vi "Set CurrSensor Record.vi"(8 "error in (no error)":errorcluster, 10 "CurrSensor":T1 {"last updated" format="%<%H:%M\n%d/%m/%Y>T"}, 11 "Main in":refnum<class "Main.lvclass">) -> (0 "error out":errorcluster, 3 "Main out":refnum<class "Main.lvclass">)   [LabVIEW 2019, in "Main.lvclass"]
uses:
  Main.lvclass
  Common/DataTypes/Sensor ranges--cluster.ctl
  Common/DataTypes/Sensor LUT--cluster.ctl
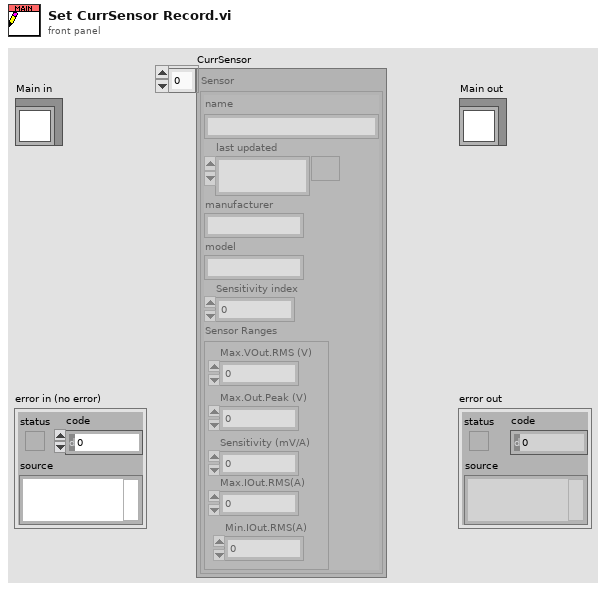
[diagram p1: front panel]
types:
  T1 = typedef "Sensor LUT--cluster.ctl" = cluster{"name":string, "last updated":timestamp, "manufacturer":string, "model":string, "Sensitivity index":dbl, "Sensor Ranges":T2}[]
  T2 = typedef "Sensor ranges--cluster.ctl" = cluster{"Max.VOut.RMS (V)":dbl, "Max.Out.Peak (V)":dbl, "Sensitivity (mV/A)":dbl, "Max.IOut.RMS(A)":dbl, "Min.IOut.RMS(A)":dbl}
  T3 = typedef "Main.lvclass/ObjData--cluster.ctl" = cluster{"Settings":T4, "Public Events":T7, "Dependency":T8, "ReadData-placeholder":T9, "VISA-placeholder":refnum<visa-resource-name>, "InverterWaveformsQ":T10, "Application.TerminateProcess Event":refnum<user-event>, "RawDaqDataQ":T11, "MeasSettings":T12, "InverterDataAcqMode":T13, "DAQState Data":T14, "Private Events":T16, "InvWfmsQ-DT":T10, "DPAuxDataQ":T17, "ProcessingState":T18, "InverterInfo":T19, "CurrInverters":T20[], "InverterLUT Dict":T24, "ESR Chart Ref":refnum<vi>[], "StoreESR BLine Ref":refnum<vi>, "UseSavedESR BLine Ref":refnum<vi>, "CurrSensor":T1}
  T4 = typedef "Main.lvclass/Settings--cluster.ctl" = cluster{"Simulation":bool, "Signal scaling":T5[], "ESR scaling":T6[], "num readings to average":i32[], "ESR alarm threshhold (%)":i32[], "UseDummyVrms":bool, "Dummy Vrms":dbl, "Inverter Database File":path, "default Inverter (name)":string[], "Minimum Current Threshold ":dbl[], "Sensors Database File":path, "default Sensors (name)":string[]}
  T5 = typedef "Main.lvclass/Gain control.ctl" = cluster{"Iin ripple gain":dbl, "Iout ripple gain":dbl, "Iout 60Hz gain ":dbl, "Vout 60Hz gain ":dbl, "Iin ripple offest":dbl, "Iout ripple offset":dbl, "Iout 60Hz offset":dbl, "Vout 60Hz offset":dbl}
  T6 = typedef "Main.lvclass/ESR scaling--cluster.ctl" = cluster{"Gain":dbl, "Offset":dbl}
  T7 = typedef "Main.lvclass/Public Events--cluster.ctl" = cluster{"Main.AsyncCmd Event":refnum<user-event>, "Main.AsyncMsg Event":refnum<user-event>, "stop process":refnum<user-event>, "UpdateControlValue Ev":refnum<user-event>, "ProcessingStateChg Ev":refnum<user-event>}
  T8 = typedef "Main.lvclass/Dependency--cluster.ctl" = cluster{"Config":refnum<class "Config.lvclass">, "DAQ":refnum<class "DAQ_Engine.lvclass">, "Log_Engine":refnum<class "Log_Engine.lvclass">}
  T9 = typedef "Main.lvclass/Read Data--cluster.ctl" = cluster{"Data":dbl}
  T10 = typedef "InverterWaveforms--QRef.ctl" = refnum<queue>
  T11 = typedef "RawDAQDataQRef--cluster.ctl" = refnum<queue>
  T12 = typedef "Measurement Config--cluster.ctl" = cluster{"Data Rate 9775":dbl, "Data Rate 9215":dbl, "Samples RMS 9215":u32, "Samples RMS 9775":u32}
  T13 = typedef "Acquisition Mode--cluster.ctl" = enum16{"3phase", "Single"}
  T14 = typedef "DAQ_Engine.lvclass/DAQStateEvData--cluster.ctl" = cluster{"DAQState":T15, "vData":variant}
  T15 = typedef "DAQState--enum.ctl" = enum16{"Unknown", "Stopped", "Running", "Error"}
  T16 = typedef "Main.lvclass/Private Events--cluster.ctl" = cluster{"PrivateAsync Ev":refnum<user-event>}
  T17 = typedef "DataProcAuxDat--Qref.ctl" = refnum<queue>
  T18 = typedef "Main.lvclass/ProcessingState--enum.ctl" = enum16{"Idle", "Starting", "Running", "Done", "Error"}
  T19 = typedef "InverterInfo--cluster.ctl" = cluster{"Inverter ID":string}
  T20 = typedef "Inverter database record v2--cluster.ctl" = cluster{"name":string, "last updated":timestamp, "type":string, "inverter Info":T21, "gain range":T22, "offset range":T23, "gain actual":dbl, "offset actual":dbl, "power level":dbl, "minimum current":dbl, "resistance single phase":dbl, "resistance 3 phase":dbl, "set flag":u16}
  T21 = typedef "inverter info v2--cluster.ctl" = cluster{"manufacturer":string, "model":string, "product":string, "serial":string, "power class":string, "year manf":string}
  T22 = typedef "inverter gain range--cluster.ctl" = cluster{"gain max":dbl, "gain min":dbl, "gain increment":dbl}
  T23 = typedef "inverter offset range--cluster.ctl" = cluster{"offset max":dbl, "offset min":dbl, "offset increment":dbl}
  T24 = typedef "TD Dynamic CVT DVR--ref.ctl" = refnum<data-value>
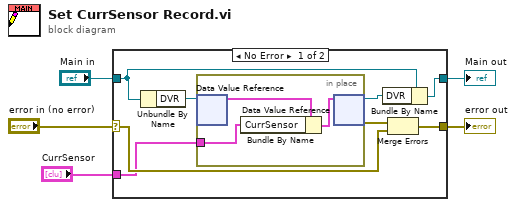
[diagram p0: block diagram]
diagram:
  n1 = case shown="No Error" "error in (no error)" {
    selector: "error in (no error)" -> [w8 w17]
    tunnel: [w7 w17] -> w4
    tunnel: [w13 w18] -> w2
    tunnel: "Main in" -> [w10 w18]
    tunnel: "CurrSensor" -> [w6 _]
    frame No Error {
      n2 = Unbundle By Name(w10) -> ("DVR"=w11:refnum<data-value>)
      n3 = in-place {
        in-place-border: w6 -> [w14]
        n4 = in-place-dvr #1(w11) -> (w16:T3)  [unwired: 1 out]
        n5 = Bundle By Name(cluster=w16, "CurrSensor"=w14) -> (w15:T3)
        n6 = in-place-dvr #1(w15) -> (w9:refnum<data-value>, w12:errorcluster)
      }
      n7 = Bundle By Name(cluster=w10, "DVR"=w9) -> (w13:refnum<class "Main.lvclass">)
      n8 = Merge Errors(w12, w8) -> (w7:errorcluster)
    }
    frame Error {
    }
  }
  "error out" <- w4
  "Main out" <- w2
